vi "Sub - window bounds to size.vi"(1 "Bounds":T1) -> (0 "Size":cluster{"Width":i16, "Height":i16})   [LabVIEW 2015, in "TLB` Template.lvlib" / "TLB`_Dependencies.lvlib"]
doc: "TLB Prime - Application Template 1.3.0.24\nNorm Kirchner, NI Systems Engineering - NI\nCopyright (c) 2014, NI"
uses:
  TLB`_Dependencies.lvlib
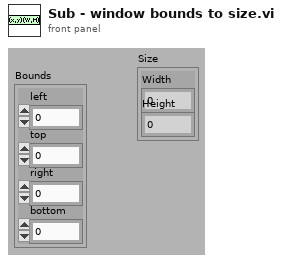
[diagram p1: front panel]
types:
  T1 = cluster{"left":i16, "top":i16, "right":i16, "bottom":i16}
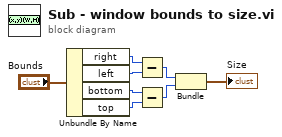
[diagram p0: block diagram]
diagram:
  n1 = Unbundle By Name("Bounds") -> ("right"=w8:i16, "left"=w7:i16, "bottom"=w6:i16, "top"=w5:i16)
  n2 = Subtract(x=w8, y=w7) -> (x-y=w4:i16)
  n3 = Subtract(x=w6, y=w5) -> (x-y=w3:i16)
  n4 = Bundle(w4, w3) -> (→"Size":cluster{i16, i16})  [unwired: 1 out]
